vi "Run.vi"(8 "error in (no error)":errorcluster caption="entrée d'erreur (pas d'erreur)", 11 "Rcv1.lvclass":refnum<class "Rcv1.lvclass">) -> (0 "error out":errorcluster caption="sortie d'erreur", 2 "Data":T1, 3 "Rcv1.lvclass":refnum<class "Rcv1.lvclass">)   [LabVIEW 2020, in "Rcv1.lvclass"]
doc: "Returns :\n\n- data : scipy csr array, dtype np.float64, shape (804414, 47236)\nThe array has 0.16% of non zero values.\n\n- target : scipy csr array, dtype np.uint8, shape (804414, 103)\nEach sample has a value of 1 in its categories, and 0 in others. The array has 3.15% of non zero values."
uses:
  Rcv1.lvclass
  Rcv1.lvclass/Rcv1.ctl
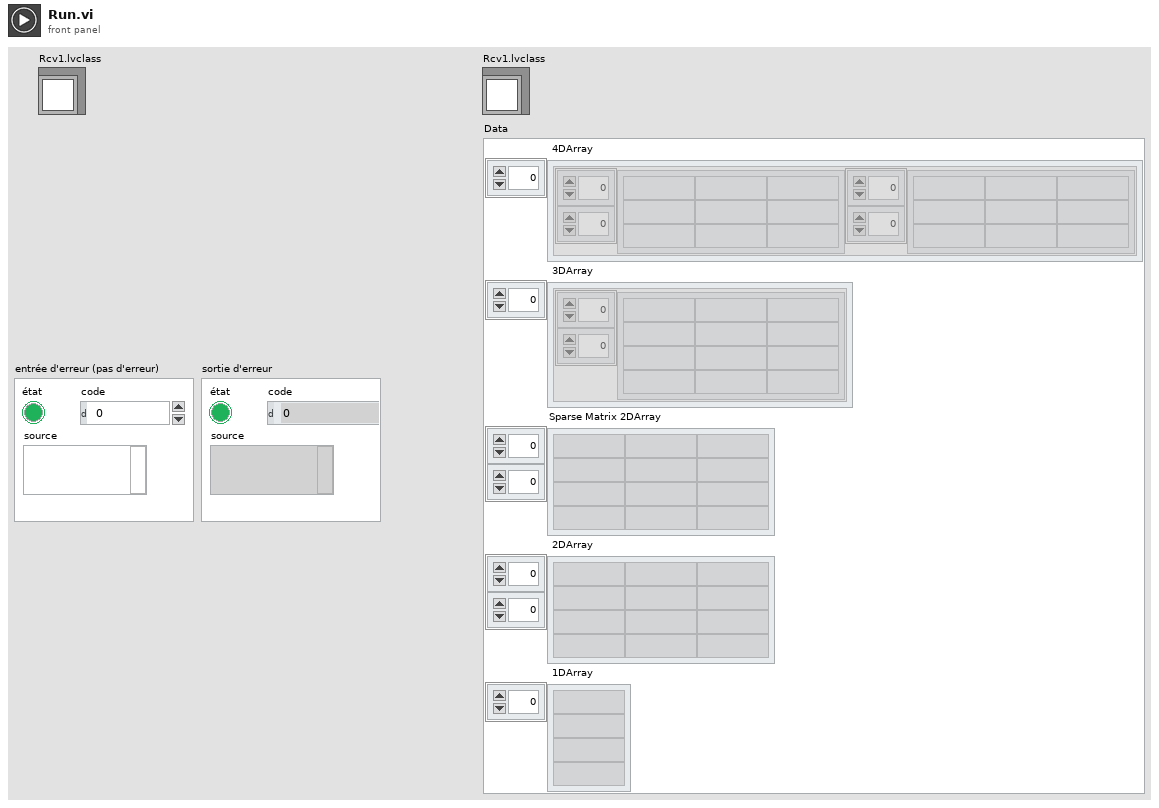
[diagram p1: front panel]
types:
  T1 = cluster{" 4DArray":cluster{"1":string[][], "2":string[][]}[], " 3DArray":cluster{"Tableau":string[][]}[], "Sparse Matrix 2DArray":string[][], " 2DArray":string[][], " 1DArray":string[]}
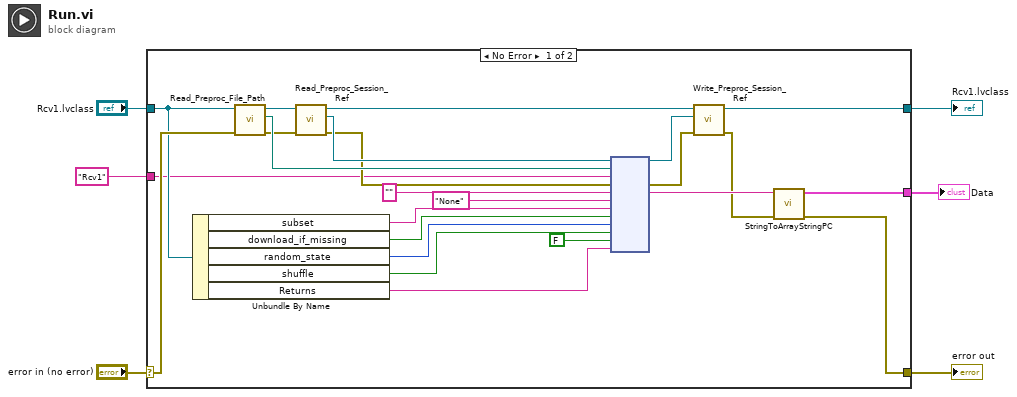
[diagram p0: block diagram]
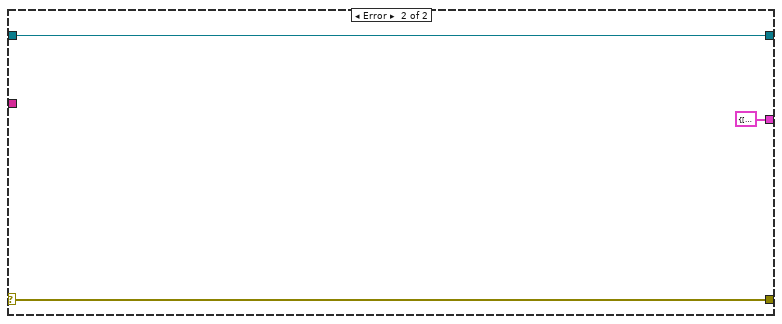
[diagram p2: hidden frame]
diagram:
  n1 = case shown="No Error" "error in (no error)" {
    selector: "error in (no error)" -> [w21 w33]
    tunnel: [w8 w33] -> w5
    tunnel: [w11 w32] -> w3
    tunnel: "Rcv1.lvclass" -> [w20 w32]
    tunnel: "Rcv1" -> [w19 _]
    tunnel: [w7 T1 {" 4DArray"=[], " 3DArray"=[], "Sparse Matrix 2DArray"=[], " 2DArray"=[], " 1DArray"=[]} ("Data")] -> w1
    frame No Error {
      n2 = Unbundle By Name(w20) -> ("subset"=w18:string, "download_if_missing"=w17:bool, "random_state"=w15:i32, "shuffle"=w14:bool, "Returns"=w12:string)
      n3 = call-dynamic "Read_Preproc_File_Path.vi"("error in (no error)"=w21, "Python in"=w20) -> ("error out"=w25:errorcluster, "File_Path"=w28:path, "Python out"=w30:refnum<class "Rcv1.lvclass">)  [unwired: 7 in]
      n4 = call-dynamic "Read_Preproc_Session_Ref.vi"("error in (no error)"=w25, "Python in"=w30) -> ("error out"=w26:errorcluster, "Session_ref"=w27:refnum<k35>, "Python out"=w29:refnum<class "Rcv1.lvclass">)  [unwired: 7 in]
      n5 = node(w27, w28, w19, w26, "", "None", w18, w17, w15, w14, FALSE, w12) -> (w22:refnum<k35>, w24:errorcluster, w10:string)  [unwired: 7 in, 2 out]
      n6 = call-dynamic "Write_Preproc_Session_Ref.vi"("error in (no error)"=w24, "Session_ref"=w22, "Python in"=w29) -> ("error out"=w9:errorcluster, "Python out"=w11:refnum<class "Rcv1.lvclass">)  [unwired: 7 in]
      n7 = call "StringToArrayStringPC.vi"("sortie d'erreur"=w9, "Return value"=w10) -> ("sortie d'erreur"=w8:errorcluster, "Data"=w7:T1)  [unwired: 8 in]
    }
    frame Error {
    }
  }
  "error out" <- w5
  "Rcv1.lvclass" <- w3
  "Data" <- w1
